vi "var_init.vi"   [LabVIEW 2018]
uses:
  examples/LABVIEW Boxman/boxman1.03.llb/global.vi
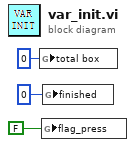
[diagram p0: block diagram]
diagram:
  n1 = global write "global.vi" "total box"(u32 0 ("total box")) -> ()
  n2 = global write "global.vi" "flag_press"(FALSE ("flag_press")) -> ()
  n3 = global write "global.vi" "finished"(u32 0 ("total box")) -> ()
